vi "Write Multiple.vi"(6 "size (unlimited)":i32, 7 "timeout in ms (-1)":i32=-1, 9 "last element? (F)":bool, 10 "elements":T1[](array[typedef])) -> (2 "channel":T2, 3 "count":i32, 4 "number unwritten":i32, 5 "timed out?":bool)   [LabVIEW 2017, in "Stream-t'WPI_EncoderType.ctl'.lvlib"]
doc: "Writes an array of elements to a Stream channel, one element at a time. The endpoint waits if the channel is full."
uses:
  <extravilib>/ChannelInstances/Stream-t'WPI_EncoderType.ctl'.lvlib
  <extravilib>/ChannelInstances/Stream-t'WPI_EncoderType.ctl'/)Channel.ctl
  <vilib>/Rock Robotics/WPI/Encoder/WPI_EncoderType.ctl
  <extravilib>/ChannelInstances/Stream-t'WPI_EncoderType.ctl'/Write With Abort.vi
  <extravilib>/ChannelInstances/Stream-t'WPI_EncoderType.ctl'/Endpoint.vi
  <resource>/ChannelSupport/_ChannelSupport/WaitIfNeeded.vi
  <extravilib>/ChannelInstances/Stream-t'WPI_EncoderType.ctl'/)Channel.vi
  <resource>/ChannelSupport/_ChannelSupport/GetErrors/FpgaChannelWireNotSupported.xnode
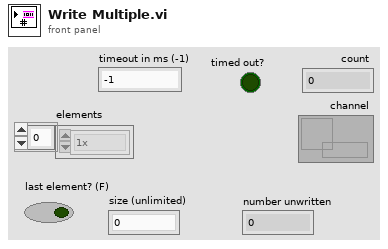
[diagram p1: front panel]
types:
  T1 = typedef "WPI_EncoderType.ctl" = enum16{"1x", "2x", "4x"}
  T2 = typedef "Stream-t'WPI_EncoderType.ctl'.lvlib/)Channel.ctl" = refnum<queue>
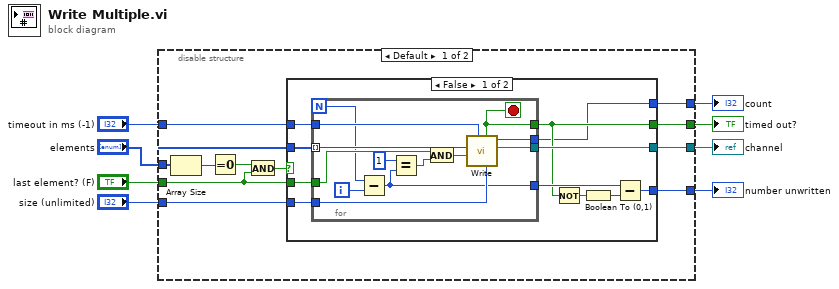
[diagram p0: block diagram]
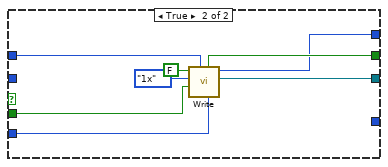
[diagram p2: hidden frame]
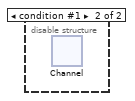
[diagram p3: hidden frame]
diagram:
  n1 = disable-structure shown="Default" {
    disable-tunnel: "size (unlimited)" -> [w19 _]
    disable-tunnel: [w18 _] -> w7
    disable-tunnel: "elements" -> [w17 _]
    disable-tunnel: "last element? (F)" -> [w13 _]
    disable-tunnel: "timeout in ms (-1)" -> [w12 _]
    disable-tunnel: [w11 _] -> w3
    disable-tunnel: [w10 _] -> w2
    disable-tunnel: [w9 _] -> w1
    frame condition #0 (active) {
      n2 = Array Size(array=w17) -> (size(s)=w16:i32)
      n3 = Equal To 0?(x=w16) -> (x = 0?=w15:bool)
      n4 = And(x=w15, y=w13) -> (x .and. y?=w14:bool)
      n5 = case shown="False" w14 {
        tunnel: w19 -> [w30 w48]
        tunnel: [w29 w51] -> w18
        tunnel: w17 -> [w28 _]
        tunnel: w13 -> [w27 w49]
        tunnel: w12 -> [w26 w46]
        tunnel: [w23 w45] -> w11
        tunnel: [w24 _] -> w10
        tunnel: [w20 w44] -> w9
        frame False {
          n6 = for {
            N -> [w35]
            tunnel: w28 -> [w40] mode=indexing
            tunnel: w30 -> [w38]
            tunnel: [w41] -> w29
            tunnel: w27 -> [w43]
            tunnel: w26 -> [w37]
            tunnel: [w36] -> w23
            tunnel: [w32] -> w25
            tunnel: [w31] -> w20
            i -> [w34]
            stop <- w36 stop-if-true
            n7 = Subtract(x=w35, y=w34) -> (x-y=w32:i32)
            n8 = Equal?(x=1, y=w32) -> (x = y?=w42:bool)
            n9 = And(x=w43, y=w42) -> (x .and. y?=w39:bool)
            n10 = call <extravilib>:"Write.vi"("size (unlimited)"=w38, "timeout in ms (-1)"=w37, "last element? (F)"=w39, "element"=w40) -> ("channel"=w41:T2, "count"=w31:i32, "timed out?"=w36:bool)  [unwired: 5 in]
          }
          n11 = Not(x=w23) -> (.not. x?=w21:bool)
          n12 = Boolean To (0,1)(Boolean=w21) -> (0, 1=w22:i16)
          n13 = Subtract(x=w25, y=w22) -> (x-y=w24:i32)
        }
        frame True {
          n14 = call <extravilib>:"Write.vi"("size (unlimited)"=w48, "timeout in ms (-1)"=w46, "last element? (F)"=w49, "element"=WPI_EncoderType."1x", "element valid? (T)"=FALSE ("valid")) -> ("channel"=w51:T2, "count"=w44:i32, "timed out?"=w45:bool)  [unwired: 4 in]
        }
      }
    }
    frame condition #1 {
      n15 = xnode "Channel"() -> ()
    }
  }
  "channel" <- w7
  "timed out?" <- w3
  "number unwritten" <- w2
  "count" <- w1
